vi "subOpenNewProject.vi"(9 "Target":string, 10 "Project path":path, 11 "BuildManager in":refnum<class "BuildManager.lvclass">) -> (0 "error out":errorcluster, 3 "BuildManager out":refnum<class "BuildManager.lvclass">)   [LabVIEW 2019, in "SolutionBuilder.lvlib" / "BuildManager.lvclass"]
uses:
  BuildManager.lvclass
  BuildManager.lvclass/BuildManager.ctl
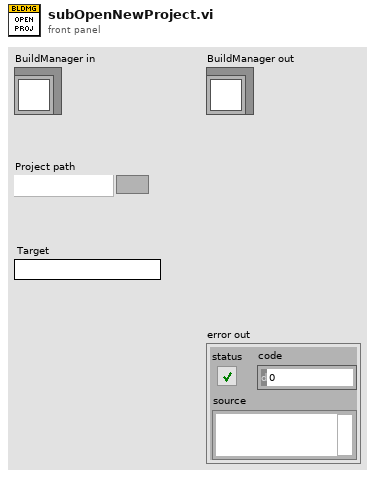
[diagram p1: front panel]
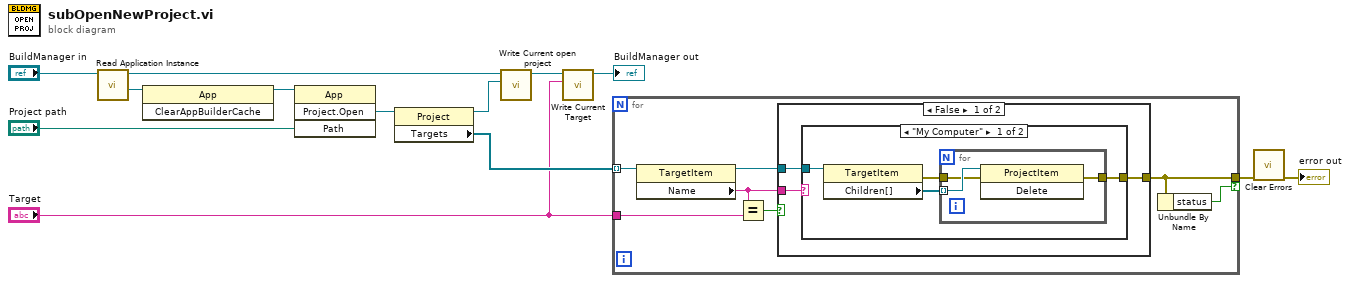
[diagram p0: block diagram]
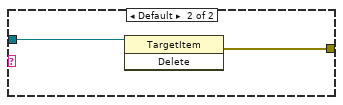
[diagram p2: hidden frame]
diagram:
  n1 = call-dynamic "Read Application Instance.vi"("BuildManager in"="BuildManager in") -> ("Application Instance"=w12:refnum<vi>, "BuildManager out"=w11:refnum<class "BuildManager.lvclass">)  [unwired: 9 in]
  n2 = invoke class="App" method="ClearAppBuilderCache"(reference=w12) -> (reference out=w13:refnum<vi>)  [unwired: 2 in, 2 out]
  n3 = invoke class="App" method="Project.Open"(reference=w13, "Path"="Project path") -> ("Project:Open"=w4:refnum<vi>)  [unwired: 2 in, 3 out]
  n4 = property class="Project"(reference=w4) -> (reference out=w3:refnum<vi>, "Targets"=w6:refnum<vi>[])  [unwired: 1 in, 1 out]
  n5 = call-dynamic "Write Current open project.vi"("Current open project"=w3, "BuildManager in"=w11) -> ("BuildManager out"=w8:refnum<class "BuildManager.lvclass">)  [unwired: 9 in]
  n6 = call "Write Current Target.vi"("Current Target"="Target", "BuildManager in"=w8) -> ("BuildManager out"=→"BuildManager out":refnum<class "BuildManager.lvclass">)  [unwired: 9 in]
  n7 = for {
    tunnel: w6 -> [w20] mode=indexing
    tunnel: "Target" -> [w19]
    tunnel: [w16] -> w2 if=w15
    n8 = property class="TargetItem"(reference=w20) -> (reference out=w18:refnum<vi>, "Name"=w14:string)  [unwired: 1 in, 1 out]
    n9 = Equal?(x=w14, y=w19) -> (x = y?=w17:bool)
    n10 = case shown="False" w17 {
      tunnel: w18 -> [w23 _]
      tunnel: [w22 _] -> w16
      tunnel: w14 -> [w21 _]
      frame False {
        n11 = case shown="\"My Computer\"" w21 {
          tunnel: w23 -> [w27 w32]
          tunnel: [w24 w31] -> w22
          frame "My Computer" {
            n12 = property class="TargetItem"(reference=w27) -> (error out=w25:errorcluster, "Children[]"=w26:refnum<vi>[])  [unwired: 1 in, 1 out]
            n13 = for {
              tunnel: w26 -> [w30] mode=indexing
              tunnel: w25 -> [w29]
              tunnel: [w28] -> w24
              n14 = invoke class="ProjectItem" method="Delete"(reference=w30, error in=w29) -> (error out=w28:errorcluster)  [unwired: 1 in, 2 out]
            }
          }
          frame Default {
            n15 = invoke class="TargetItem" method="Delete"(reference=w32) -> (error out=w31:errorcluster)  [unwired: 2 in, 2 out]
          }
        }
      }
      frame True {
      }
    }
    n16 = Unbundle By Name(w16) -> ("status"=w15:bool)
  }
  n17 = call <vilib>:"Clear Errors.vi"("error in (no error)"=w2) -> ("error out"=→"error out":errorcluster)  [unwired: 5 in, 1 out]
